vi "Check Color Range Ball.vi"(11 "Ball Color Range":refnum<vi>) -> ()   [LabVIEW 2023]
uses:
  <vilib>/Rock Robotics/Network Tables/NT Read String.vi
  <vilib>/Rock Robotics/Network Tables/NT Write String.vi
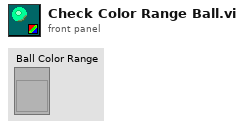
[diagram p1: front panel]
types:
  T1 = cluster{"Hue":cluster{dbl, dbl}, "Sat":cluster{dbl, dbl}, "Val":cluster{dbl, dbl}}
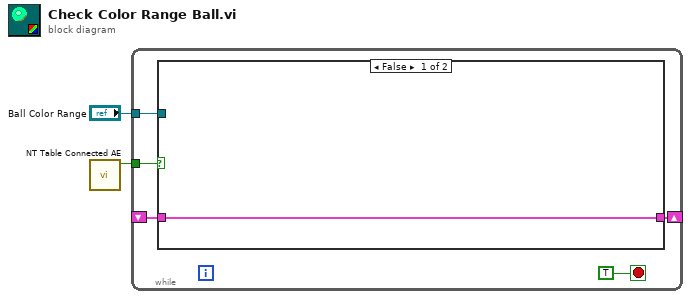
[diagram p0: block diagram]
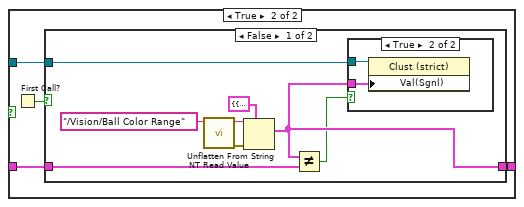
[diagram p2: hidden frame]
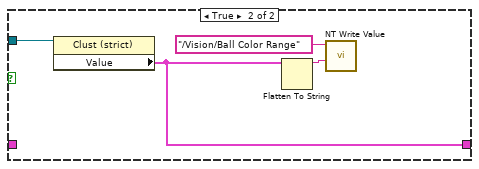
[diagram p4: hidden frame]
diagram:
  n1 = call "NT Table Connected AE.vi"() -> ("NT Table Connected out"=w1:bool)  [unwired: 11 in]
  n2 = while {
    shift-right: [w5] -> _
    shift-left: _ -> [w6]
    tunnel: "Ball Color Range" -> [w4]
    tunnel: w1 -> [w3]
    stop <- TRUE stop-if-true
    n3 = case shown="False" w3 {
      tunnel: w6 -> [w8 w12]
      tunnel: [w8 w11] -> w5
      tunnel: w4 -> [_ w10]
      frame False {
      }
      frame True {
        n4 = First Call?() -> (First Call?: T/F=w9:bool)
        n5 = case shown="False" w9 {
          tunnel: w12 -> [w17 _]
          tunnel: [w16 w23] -> w11
          tunnel: w10 -> [w13 w26]
          frame False {
            n6 = call-poly <vilib>:"NT Read Value.vi"("name"="/Vision/Ball Color Range" ("Name")) -> ("error out"=w18:errorcluster, "value"=w19:string)  [unwired: 8 in, 1 out]
            n7 = Unflatten From String(type=T1 {"Hue"={103.0, 151.0}, "Sat"={216.98804569244385, 255.0}, "Val"={201.0, 249.0}} ("Port Color Range"), binary string=w19, error in (no error)=w18) -> (value=w16:T1)  [unwired: 2 in, 2 out]
            n8 = Not Equal?(x=w16, y=w17) -> (x != y?=w15:bool)
            n9 = case shown="True" w15 {
              tunnel: w13 -> [_ w22]
              tunnel: w16 -> [_ w21]
              frame False {
              }
              frame True {
                n10 = property on="Property Node" class="Clust (strict)"(reference=w22, "Val(Sgnl)"=w21) -> ()  [unwired: 1 in, 2 out]
              }
            }
          }
          frame True {
            n11 = property class="Clust (strict)"(reference=w26) -> ("Value"=w23:T1)  [unwired: 1 in, 2 out]
            n12 = Flatten To String(anything=w23) -> (data string=w25:string)  [unwired: 3 in, 2 out]
            n13 = call-poly <vilib>:"NT Write Value.vi"("value"=w25, "name"="/Vision/Ball Color Range" ("Name")) -> ()  [unwired: 9 in, 1 out]
          }
        }
      }
    }
  }
